vi "Lab Panel V4.85.vi"() -> ()   [LabVIEW 2013] (continued)
                    n2580 = Unbundle(w4668) -> ("DESCRIPTION"=w4648:string)  [unwired: 4 out]
                    n2581 = Unbundle(w4667) -> ("DESCRIPTION"=w4647:string)  [unwired: 4 out]
                    n2582 = Unbundle(w4664) -> ("DESCRIPTION"=w4644:string)  [unwired: 4 out]
                    n2583 = Unbundle(w4670) -> ("DESCRIPTION"=w4650:string)  [unwired: 4 out]
                    n2584 = Unbundle(w4666) -> ("DESCRIPTION"=w4646:string)  [unwired: 4 out]
                    n2585 = Unbundle(w4673) -> ("DESCRIPTION"=w4662:string)  [unwired: 4 out]
                    n2586 = Unbundle(w4671) -> ("DESCRIPTION"=w4651:string)  [unwired: 4 out]
                    n2587 = Unbundle(w4665) -> ("DESCRIPTION"=w4645:string)  [unwired: 4 out]
                    n2588 = Unbundle(w4672) -> ("DESCRIPTION"=w4652:string)  [unwired: 4 out]
                    n2589 = Concatenate Strings("[LAB05-2/", w4644) -> (w4634:string)
                    n2590 = Concatenate Strings("[LAB05-1/", w4645) -> (w4635:string)
                    n2591 = Concatenate Strings("[LAB04-2/", w4646) -> (w4636:string)
                    n2592 = Concatenate Strings("[LAB03-2/", w4648) -> (w4638:string)
                    n2593 = Concatenate Strings("[LAB04-1/", w4647) -> (w4637:string)
                    n2594 = Concatenate Strings("[LAB03-1/", w4649) -> (w4639:string)
                    n2595 = Concatenate Strings("[LAB01-2/", w4652) -> (w4642:string)
                    n2596 = Concatenate Strings("[LAB02-2/", w4650) -> (w4640:string)
                    n2597 = Concatenate Strings("[LAB01-1/", w4662) -> (w4643:string)
                    n2598 = Concatenate Strings("[LAB02-1/", w4651) -> (w4641:string)
                  }
                  frame #1 {
                    w4697 = "/"
                    w4698 = 2.0
                    n2599 = local read "DISP LAB01-2"() -> (w4777:T4)
                    n2600 = local read "DISP LAB01-1"() -> (w4778:T4)
                    n2601 = local read "DISP LAB02-1"() -> (w4776:T4)
                    n2602 = local read "DISP LAB03-2"() -> (w4773:T4)
                    n2603 = local read "DISP LAB02-2"() -> (w4775:T4)
                    n2604 = local read "DISP LAB03-1"() -> (w4774:T4)
                    n2605 = local read "DISP LAB04-2"() -> (w4771:T4)
                    n2606 = local read "DISP LAB04-1"() -> (w4772:T4)
                    n2607 = local read "DISP LAB05-1"() -> (w4770:T4)
                    n2608 = local read "DISP LAB05-2"() -> (w4769:T4)
                    n2609 = Unbundle(w4777) -> ("CYCLE"=w4761:dbl, "MINS"=w4760:dbl, "STATUS"=w4757:string)
                    n2610 = Unbundle(w4778) -> ("CYCLE"=w4766:dbl, "MINS"=w4765:dbl, "STATUS"=w4762:string)
                    n2611 = Unbundle(w4776) -> ("CYCLE"=w4754:dbl, "MINS"=w4753:dbl, "STATUS"=w4752:string)
                    n2612 = Unbundle(w4773) -> ("CYCLE"=w4741:dbl, "MINS"=w4740:dbl, "STATUS"=w4737:string)
                    n2613 = Unbundle(w4774) -> ("CYCLE"=w4746:dbl, "MINS"=w4745:dbl, "STATUS"=w4742:string)
                    n2614 = Unbundle(w4775) -> ("CYCLE"=w4751:dbl, "MINS"=w4750:dbl, "STATUS"=w4747:string)
                    n2615 = Unbundle(w4772) -> ("CYCLE"=w4736:dbl, "MINS"=w4735:dbl, "STATUS"=w4732:string)
                    n2616 = Unbundle(w4771) -> ("CYCLE"=w4731:dbl, "MINS"=w4730:dbl, "STATUS"=w4727:string)
                    n2617 = Unbundle(w4770) -> ("CYCLE"=w4726:dbl, "MINS"=w4725:dbl, "STATUS"=w4722:string)
                    n2618 = Unbundle(w4769) -> ("CYCLE"=w4768:dbl, "MINS"=w4767:dbl, "STATUS"=w4719:string)
                    n2619 = Number To Decimal String(number=w4754) -> (decimal integer string=w4756:string)  [unwired: 1 in]
                    n2620 = Number To Decimal String(number=w4751) -> (decimal integer string=w4749:string)  [unwired: 1 in]
                    n2621 = Number To Decimal String(number=w4746) -> (decimal integer string=w4744:string)  [unwired: 1 in]
                    n2622 = Number To Decimal String(number=w4761) -> (decimal integer string=w4759:string)  [unwired: 1 in]
                    n2623 = Number To Decimal String(number=w4741) -> (decimal integer string=w4739:string)  [unwired: 1 in]
                    n2624 = Number To Decimal String(number=w4766) -> (decimal integer string=w4764:string)  [unwired: 1 in]
                    n2625 = Number To Decimal String(number=w4768) -> (decimal integer string=w4721:string)  [unwired: 1 in]
                    n2626 = Number To Decimal String(number=w4736) -> (decimal integer string=w4734:string)  [unwired: 1 in]
                    n2627 = Number To Decimal String(number=w4731) -> (decimal integer string=w4729:string)  [unwired: 1 in]
                    n2628 = Number To Decimal String(number=w4726) -> (decimal integer string=w4724:string)  [unwired: 1 in]
                    n2629 = Number To Fractional String(number=w4753, precision (6)=w4698) -> (F-format string=w4755:string)  [unwired: 2 in]
                    n2630 = Number To Fractional String(number=w4740, precision (6)=w4698) -> (F-format string=w4738:string)  [unwired: 2 in]
                    n2631 = Number To Fractional String(number=w4750, precision (6)=w4698) -> (F-format string=w4748:string)  [unwired: 2 in]
                    n2632 = Number To Fractional String(number=w4745, precision (6)=w4698) -> (F-format string=w4743:string)  [unwired: 2 in]
                    n2633 = Number To Fractional String(number=w4730, precision (6)=w4698) -> (F-format string=w4728:string)  [unwired: 2 in]
                    n2634 = Number To Fractional String(number=w4735, precision (6)=w4698) -> (F-format string=w4733:string)  [unwired: 2 in]
                    n2635 = Number To Fractional String(number=w4760, precision (6)=w4698) -> (F-format string=w4758:string)  [unwired: 2 in]
                    n2636 = Number To Fractional String(number=w4725, precision (6)=w4698) -> (F-format string=w4723:string)  [unwired: 2 in]
                    n2637 = Number To Fractional String(number=w4765, precision (6)=w4698) -> (F-format string=w4763:string)  [unwired: 2 in]
                    n2638 = Number To Fractional String(number=w4767, precision (6)=w4698) -> (F-format string=w4720:string)  [unwired: 2 in]
                    n2639 = Concatenate Strings(w4697, w4739, w4697, w4738, w4697, w4737) -> (w4713:string)
                    n2640 = Concatenate Strings(w4697, w4734, w4697, w4733, w4697, w4732) -> (w4712:string)
                    n2641 = Concatenate Strings(w4697, w4729, w4697, w4728, w4697, w4727) -> (w4711:string)
                    n2642 = Concatenate Strings(w4697, w4724, w4697, w4723, w4697, w4722) -> (w4710:string)
                    n2643 = Concatenate Strings(w4697, w4721, w4697, w4720, w4697, w4719) -> (w4709:string)
                    n2644 = Concatenate Strings(w4697, w4764, w4697, w4763, w4697, w4762) -> (w4718:string)
                    n2645 = Concatenate Strings(w4697, w4744, w4697, w4743, w4697, w4742) -> (w4714:string)
                    n2646 = Concatenate Strings(w4697, w4759, w4697, w4758, w4697, w4757) -> (w4717:string)
                    n2647 = Concatenate Strings(w4697, w4756, w4697, w4755, w4697, w4752) -> (w4716:string)
                    n2648 = Concatenate Strings(w4697, w4749, w4697, w4748, w4697, w4747) -> (w4715:string)
                    n2649 = Concatenate Strings("]", "\r") -> (w4694:string)
                    n2650 = Concatenate Strings(w4689, w4714, w4694) -> (w4704:string)
                    n2651 = Concatenate Strings(w4691, w4716, w4694) -> (w4706:string)
                    n2652 = Concatenate Strings(w4690, w4715, w4694) -> (w4705:string)
                    n2653 = Concatenate Strings(w4686, w4711, w4694) -> (w4701:string)
                    n2654 = Concatenate Strings(w4687, w4710, w4694) -> (w4702:string)
                    n2655 = Concatenate Strings(w4685, w4712, w4694) -> (w4700:string)
                    n2656 = Concatenate Strings(w4684, w4713, w4694) -> (w4699:string)
                    n2657 = Concatenate Strings(w4688, w4709, w4694) -> (w4703:string)
                    n2658 = Concatenate Strings(w4692, w4717, w4694) -> (w4707:string)
                    n2659 = Concatenate Strings(w4693, w4718, w4694) -> (w4708:string)
                    n2660 = Concatenate Strings(w4708, w4707, w4706, w4705, w4704, w4699, w4700, w4701, w4702, w4703) -> (w4677:string)
                    n2661 = Concatenate Strings("[PANEL/", "DESC/", "CYCLES/", "MINS/", "STATUS]", "\r", w4677) -> (w4676:string)
                    "MAIL REPORT" <- w4676
                    n2662 = global write "Global display 3.vi" "log all"(w4676) -> ()
                  }
                  frame #2 {
                    w4807 = "END"
                    n2663 = local read "mail control"() -> (w4808:string)
                    n2664 = case shown="False" w4803 {
                      tunnel: w4808 -> [w4832 _]
                      tunnel: w4807 -> [w4831 _]
                      tunnel: [w4830 FALSE] -> w4793
                      frame False {
                        n2665 = Equal?(x=w4832, y=w4831) -> (x = y?=w4830:bool)
                      }
                      frame True {
                      }
                    }
                    n2666 = case shown="False" w4809 {
                      tunnel: w4808 -> [w4848 _]
                      tunnel: w4807 -> [w4847 _]
                      tunnel: [w4846 FALSE] -> w4797
                      frame False {
                        n2667 = Equal?(x=w4848, y=w4847) -> (x = y?=w4846:bool)
                      }
                      frame True {
                      }
                    }
                    n2668 = case shown="False" w4806 {
                      tunnel: w4808 -> [w4844 _]
                      tunnel: w4807 -> [w4843 _]
                      tunnel: [w4842 FALSE] -> w4796
                      frame False {
                        n2669 = Equal?(x=w4844, y=w4843) -> (x = y?=w4842:bool)
                      }
                      frame True {
                      }
                    }
                    n2670 = case shown="False" w4804 {
                      tunnel: w4808 -> [w4836 _]
                      tunnel: w4807 -> [w4835 _]
                      tunnel: [w4834 FALSE] -> w4794
                      frame False {
                        n2671 = Equal?(x=w4836, y=w4835) -> (x = y?=w4834:bool)
                      }
                      frame True {
                      }
                    }
                    n2672 = case shown="False" w4805 {
                      tunnel: w4808 -> [w4840 _]
                      tunnel: w4807 -> [w4839 _]
                      tunnel: [w4838 FALSE] -> w4795
                      frame False {
                        n2673 = Equal?(x=w4840, y=w4839) -> (x = y?=w4838:bool)
                      }
                      frame True {
                      }
                    }
                    n2674 = Or(x=w4795, y=w4794) -> (x .or. y?=w4786:bool)
                    n2675 = Or(x=w4797, y=w4796) -> (x .or. y?=w4787:bool)
                    n2676 = Or(x=w4787, y=w4786) -> (x .or. y?=w4782:bool)
                    n2677 = case shown="False" w4799 {
                      tunnel: w4808 -> [w4816 _]
                      tunnel: w4807 -> [w4815 _]
                      tunnel: [w4814 FALSE] -> w4788
                      frame False {
                        n2678 = Equal?(x=w4816, y=w4815) -> (x = y?=w4814:bool)
                      }
                      frame True {
                      }
                    }
                    n2679 = case shown="False" w4798 {
                      tunnel: w4808 -> [w4812 _]
                      tunnel: w4807 -> [w4811 _]
                      tunnel: [w4810 FALSE] -> w4792
                      frame False {
                        n2680 = Equal?(x=w4812, y=w4811) -> (x = y?=w4810:bool)
                      }
                      frame True {
                      }
                    }
                    n2681 = case shown="False" w4800 {
                      tunnel: w4808 -> [w4820 _]
                      tunnel: w4807 -> [w4819 _]
                      tunnel: [w4818 FALSE] -> w4789
                      frame False {
                        n2682 = Equal?(x=w4820, y=w4819) -> (x = y?=w4818:bool)
                      }
                      frame True {
                      }
                    }
                    n2683 = case shown="False" w4802 {
                      tunnel: w4808 -> [w4828 _]
                      tunnel: w4807 -> [w4827 _]
                      tunnel: [w4826 FALSE] -> w4791
                      frame False {
                        n2684 = Equal?(x=w4828, y=w4827) -> (x = y?=w4826:bool)
                      }
                      frame True {
                      }
                    }
                    n2685 = case shown="False" w4801 {
                      tunnel: w4808 -> [w4824 _]
                      tunnel: w4807 -> [w4823 _]
                      tunnel: [w4822 FALSE] -> w4790
                      frame False {
                        n2686 = Equal?(x=w4824, y=w4823) -> (x = y?=w4822:bool)
                      }
                      frame True {
                      }
                    }
                    n2687 = Or(x=w4791, y=w4790) -> (x .or. y?=w4785:bool)
                    n2688 = Or(x=w4789, y=w4788) -> (x .or. y?=w4784:bool)
                    n2689 = Or(x=w4792, y=w4793) -> (x .or. y?=w4780:bool)
                    n2690 = Or(x=w4785, y=w4784) -> (x .or. y?=w4783:bool)
                    n2691 = Or(x=w4782, y=w4783) -> (x .or. y?=w4781:bool)
                    n2692 = Or(x=w4781, y=w4780) -> (x .or. y?=w4779:bool)
                  }
                  frame #3 {
                    n2693 = local read "on loops"() -> (w4862:dbl)
                    n2694 = local read "jig cycle"() -> (w4859:dbl)
                    n2695 = local read "Send Mail Now"() -> (w4853:bool)
                    n2696 = Add(x=w4862, y=3.0) -> (x+y=w4860:dbl)
                    n2697 = Equal?(x=w4859, y=w4860) -> (x = y?=w4854:bool)
                    n2698 = And(x=w4854, y=w4853) -> (x .and. y?=w4852:bool)
                    n2699 = And(x=w4858, y=w4854) -> (x .and. y?=w4857:bool)
                    n2700 = And(x=w4857, y=w4856) -> (x .and. y?=w4855:bool)
                    n2701 = Or(x=w4855, y=w4852) -> (x .or. y?=w4851:bool)
                    n2702 = case shown="True" w4851 {
                      tunnel: w4867 -> [_ w4873]
                      tunnel: w4866 -> [_ w4872]
                      tunnel: "Lab Panel Test Status" -> [_ w4871]
                      tunnel: w4864 -> [_ w4870]
                      tunnel: w4863 -> [_ w4869]
                      tunnel: w4850 -> [_ w4868]
                      frame False {
                      }
                      frame True {
                        n2703 = stacked-sequence {
                          tunnel: w4873 -> [w4881 _]
                          tunnel: w4872 -> [w4880 _]
                          tunnel: w4871 -> [w4879 _]
                          tunnel: w4870 -> [w4878 _]
                          tunnel: w4869 -> [w4877 _]
                          tunnel: w4868 -> [w4876 _]
                          frame #0 {
                            n2704 = call "sub vi - send mail v5.vi"("TO:"=w4881, "subject"=w4879, "from"=w4877, "out going server"=w4878, "message"=w4880) -> ("error out"=w4875:errorcluster)  [unwired: 10 in]
                            n2705 = Bundle(cluster=w4876, "mail error"=w4875) -> (w4874:T6)  [unwired: 6 in]
                            n2706 = local write "MAIL SETTINGS"(w4874) -> ()
                          }
                          frame #1 {
                            n2707 = local write "mail control"("") -> ()
                            n2708 = local write "Send Mail Now"(FALSE) -> ()
                          }
                        }
                      }
                    }
                  }
                }
              }
            }
          }
          frame #18 {
            # "save jig cycle values once all run switches are off"
            n2709 = stacked-sequence {
              tunnel: w4893 -> [_ w4922]
              tunnel: w4892 -> [_ w4921]
              tunnel: w4891 -> [_ w4920]
              tunnel: w4890 -> [_ w4919]
              tunnel: w4889 -> [_ w4918]
              tunnel: w4888 -> [_ w4917]
              tunnel: w4887 -> [_ w4916]
              tunnel: w4886 -> [_ w4915]
              tunnel: w4885 -> [_ w4914]
              tunnel: w4884 -> [_ w4913]
              frame #0 {
              }
              frame #1 {
                n2710 = Not(x=w4913) -> (.not. x?=w4896:bool)
                n2711 = Not(x=w4921) -> (.not. x?=w4911:bool)
                n2712 = Not(x=w4918) -> (.not. x?=w4906:bool)
                n2713 = Not(x=w4916) -> (.not. x?=w4902:bool)
                n2714 = Not(x=w4914) -> (.not. x?=w4898:bool)
                n2715 = Not(x=w4922) -> (.not. x?=w4912:bool)
                n2716 = Not(x=w4920) -> (.not. x?=w4910:bool)
                n2717 = Not(x=w4917) -> (.not. x?=w4904:bool)
                n2718 = Not(x=w4919) -> (.not. x?=w4908:bool)
                n2719 = Not(x=w4915) -> (.not. x?=w4900:bool)
                n2720 = local read "Save JC"() -> (w4924:bool)
                n2721 = And(x=w4912, y=w4911) -> (x .and. y?=w4909:bool)
                n2722 = And(x=w4909, y=w4910) -> (x .and. y?=w4907:bool)
                n2723 = And(x=w4907, y=w4908) -> (x .and. y?=w4905:bool)
                n2724 = And(x=w4905, y=w4906) -> (x .and. y?=w4903:bool)
                n2725 = And(x=w4903, y=w4904) -> (x .and. y?=w4901:bool)
                n2726 = And(x=w4901, y=w4902) -> (x .and. y?=w4899:bool)
                n2727 = And(x=w4899, y=w4900) -> (x .and. y?=w4897:bool)
                n2728 = And(x=w4897, y=w4898) -> (x .and. y?=w4895:bool)
                n2729 = And(x=w4895, y=w4896) -> (x .and. y?=w4894:bool)
                n2730 = And(x=w4894, y=w4924) -> (x .and. y?=w4923:bool)
                n2731 = case shown="True" w4923 {
                  tunnel: w4894 -> [w4925 _]
                  frame False {
                    n2732 = case shown="False" w4925 {
                      frame False {
                        n2733 = local write "Save JC"(TRUE) -> ()
                      }
                      frame True {
                      }
                    }
                  }
                  frame True {
                    n2734 = stacked-sequence {
                      frame #0 {
                        n2735 = String To Path(string="c:\\crabtree\\Jig Cycles\\") -> (path=w4937:path)
                        n2736 = Build Path(base path=w4937, name or relative path="jigcycles.bin") -> (appended path=w4935:path)
                        n2737 = Create Folder(path (use dialog)=w4937) -> (error out=w4939:errorcluster)  [unwired: 2 in, 2 out]
                        n2738 = local read "JIG RELAY CYCLES"() -> (w4929:T7)
                        n2739 = call <vilib>:"Clear Errors.vi"("error in (no error)"=w4939) -> ()  [unwired: 6 in, 1 out]
                        n2740 = local write "Save JC"(FALSE) -> ()
                        n2741 = Open/Create/Replace File(file path (use dialog)=w4935, operation (0:open)=T19."replace or create") -> (refnum out=w4933:refnum<file>, error out=w4934:errorcluster)  [unwired: 4 in, 1 out]
                        n2742 = Write to Binary File(file (use dialog)=w4933, data=w4929, error in=w4934) -> (refnum out=w4932:refnum<file>, error out=w4931:errorcluster)  [unwired: 3 in, 1 out]
                        n2743 = Close File(refnum=w4932, error in=w4931) -> (error out=w4930:errorcluster)  [unwired: 1 out]
                        n2744 = local write "data file error"(w4930) -> ()
                      }
                      frame #1 {
                        n2745 = local read "JIG RELAY CYCLES"() -> (w4962:T7)
                        n2746 = Unbundle By Name(w4962) -> ("LAB01-1"=w4957:dbl, "LAB01-2"=w4956:dbl, "LAB02-1"=w4954:dbl, "LAB02-2"=w4953:dbl, "LAB03-1"=w4951:dbl, "LAB03-2"=w4948:dbl, "LAB04-1"=w4947:dbl, "LAB04-2"=w4945:dbl, "LAB05-1"=w4943:dbl, "LAB05-2"=w4941:dbl)
                        n2747 = stacked-sequence {
                          tunnel: w4957 -> [w4965 _ _ _ _ _ _ _ _ _]
                          tunnel: 1000000 -> [w4968 w4978 w4988 w4998 w5008 w5018 w5028 w5038 w5048 w5058]
                          tunnel: [w4966 _ _ _ _ _ _ _ _ _] -> w4960
                          tunnel: "TEST STATION HAS REACHED 1 MILLION CYCLES, REPLACE  CONTROL RELAYS" -> [w4964 w4976 w4986 w4996 w5006 w5016 w5026 w5036 w5046 w5056]
                          tunnel: [_ w4975 _ _ _ _ _ _ _ _] -> w4958
                          tunnel: w4956 -> [_ w4974 _ _ _ _ _ _ _ _]
                          tunnel: [_ _ w4985 _ _ _ _ _ _ _] -> w4955
                          tunnel: w4954 -> [_ _ w4984 _ _ _ _ _ _ _]
                          tunnel: w4953 -> [_ _ _ w4995 _ _ _ _ _ _]
                          tunnel: [_ _ _ w4994 _ _ _ _ _ _] -> w4952
                          tunnel: w4951 -> [_ _ _ _ w5005 _ _ _ _ _]
                          tunnel: [_ _ _ _ w5004 _ _ _ _ _] -> w4950
                          tunnel: [_ _ _ _ _ w5015 _ _ _ _] -> w4949
                          tunnel: w4948 -> [_ _ _ _ _ w5014 _ _ _ _]
                          tunnel: w4947 -> [_ _ _ _ _ _ w5025 _ _ _]
                          tunnel: [_ _ _ _ _ _ w5024 _ _ _] -> w4946
                          tunnel: w4945 -> [_ _ _ _ _ _ _ w5035 _ _]
                          tunnel: [_ _ _ _ _ _ _ w5034 _ _] -> w4944
                          tunnel: w4943 -> [_ _ _ _ _ _ _ _ w5045 _]
                          tunnel: [_ _ _ _ _ _ _ _ w5044 _] -> w4942
                          tunnel: w4941 -> [_ _ _ _ _ _ _ _ _ w5055]
                          tunnel: [_ _ _ _ _ _ _ _ _ w5054] -> w4940
                          frame #0 {
                            n2748 = Greater?(x=w4965, y=w4968) -> (0:w4967:bool)
                            n2749 = case shown="True" w4967 {
                              tunnel: [w4969 0] -> w4966
                              tunnel: w4965 -> [w4969 _]
                              tunnel: w4964 -> [_ w4970]
                              frame False {
                              }
                              frame True {
                                n2750 = Concatenate Strings("LA01-1 ", w4970) -> (w4973:string)
                                n2751 = One Button Dialog(message=w4973) -> ()  [unwired: 1 in, 1 out]
                              }
                            }
                          }
                          frame #1 {
                            n2752 = Greater?(x=w4974, y=w4978) -> (0:w4977:bool)
                            n2753 = case shown="True" w4977 {
                              tunnel: [w4979 0] -> w4975
                              tunnel: w4974 -> [w4979 _]
                              tunnel: w4976 -> [_ w4980]
                              frame False {
                              }
                              frame True {
                                n2754 = Concatenate Strings("LA01-2 ", w4980) -> (w4983:string)
                                n2755 = One Button Dialog(message=w4983) -> ()  [unwired: 1 in, 1 out]
                              }
                            }
                          }
                          frame #2 {
                            n2756 = Greater?(x=w4984, y=w4988) -> (0:w4987:bool)
                            n2757 = case shown="True" w4987 {
                              tunnel: [w4989 0] -> w4985
                              tunnel: w4984 -> [w4989 _]
                              tunnel: w4986 -> [_ w4990]
                              frame False {
                              }
                              frame True {
                                n2758 = Concatenate Strings("LA02-1 ", w4990) -> (w4993:string)
                                n2759 = One Button Dialog(message=w4993) -> ()  [unwired: 1 in, 1 out]
                              }
                            }
                          }
                          frame #3 {
                            n2760 = Greater?(x=w4995, y=w4998) -> (0:w4997:bool)
                            n2761 = case shown="True" w4997 {
                              tunnel: [w4999 0] -> w4994
                              tunnel: w4995 -> [w4999 _]
                              tunnel: w4996 -> [_ w5000]
                              frame False {
                              }
                              frame True {
                                n2762 = Concatenate Strings("LA02-2 ", w5000) -> (w5003:string)
                                n2763 = One Button Dialog(message=w5003) -> ()  [unwired: 1 in, 1 out]
                              }
                            }
                          }
                          frame #4 {
                            n2764 = Greater?(x=w5005, y=w5008) -> (0:w5007:bool)
                            n2765 = case shown="True" w5007 {
                              tunnel: [w5009 0] -> w5004
                              tunnel: w5005 -> [w5009 _]
                              tunnel: w5006 -> [_ w5010]
                              frame False {
                              }
                              frame True {
                                n2766 = Concatenate Strings("LA03-1 ", w5010) -> (w5013:string)
                                n2767 = One Button Dialog(message=w5013) -> ()  [unwired: 1 in, 1 out]
                              }
                            }
                          }
                          frame #5 {
                            n2768 = Greater?(x=w5014, y=w5018) -> (0:w5017:bool)
                            n2769 = case shown="True" w5017 {
                              tunnel: [w5019 0] -> w5015
                              tunnel: w5014 -> [w5019 _]
                              tunnel: w5016 -> [_ w5020]
                              frame False {
                              }
                              frame True {
                                n2770 = Concatenate Strings("LA03-2 ", w5020) -> (w5023:string)
                                n2771 = One Button Dialog(message=w5023) -> ()  [unwired: 1 in, 1 out]
                              }
                            }
                          }
                          frame #6 {
                            n2772 = Greater?(x=w5025, y=w5028) -> (0:w5027:bool)
                            n2773 = case shown="True" w5027 {
                              tunnel: [w5029 0] -> w5024
                              tunnel: w5025 -> [w5029 _]
                              tunnel: w5026 -> [_ w5030]
                              frame False {
                              }
                              frame True {
                                n2774 = Concatenate Strings("LA04-1 ", w5030) -> (w5033:string)
                                n2775 = One Button Dialog(message=w5033) -> ()  [unwired: 1 in, 1 out]
                              }
                            }
                          }
                          frame #7 {
                            n2776 = Greater?(x=w5035, y=w5038) -> (0:w5037:bool)
                            n2777 = case shown="True" w5037 {
                              tunnel: [w5039 0] -> w5034
                              tunnel: w5035 -> [w5039 _]
                              tunnel: w5036 -> [_ w5040]
                              frame False {
                              }
                              frame True {
                                n2778 = Concatenate Strings("LA04-2 ", w5040) -> (w5043:string)
                                n2779 = One Button Dialog(message=w5043) -> ()  [unwired: 1 in, 1 out]
                              }
                            }
                          }
                          frame #8 {
                            n2780 = Greater?(x=w5045, y=w5048) -> (0:w5047:bool)
                            n2781 = case shown="True" w5047 {
                              tunnel: [w5049 0] -> w5044
                              tunnel: w5045 -> [w5049 _]
                              tunnel: w5046 -> [_ w5050]
                              frame False {
                              }
                              frame True {
                                n2782 = Concatenate Strings("LA05-1 ", w5050) -> (w5053:string)
                                n2783 = One Button Dialog(message=w5053) -> ()  [unwired: 1 in, 1 out]
                              }
                            }
                          }
                          frame #9 {
                            n2784 = Greater?(x=w5055, y=w5058) -> (0:w5057:bool)
                            n2785 = case shown="True" w5057 {
                              tunnel: [w5059 0] -> w5054
                              tunnel: w5055 -> [w5059 _]
                              tunnel: w5056 -> [_ w5060]
                              frame False {
                              }
                              frame True {
                                n2786 = Concatenate Strings("LA05-2 ", w5060) -> (w5063:string)
                                n2787 = One Button Dialog(message=w5063) -> ()  [unwired: 1 in, 1 out]
                              }
                            }
                          }
                        }
                        n2788 = Bundle By Name(cluster=w4962, "LAB01-1"=w4960, "LAB01-2"=w4958, "LAB02-1"=w4955, "LAB02-2"=w4952, "LAB03-1"=w4950, "LAB03-2"=w4949, "LAB04-1"=w4946, "LAB04-2"=w4944, "LAB05-1"=w4942, "LAB05-2"=w4940) -> (w4961:T7)
                        n2789 = local write "JIG RELAY CYCLES"(w4961) -> ()
                      }
                    }
                  }
                }
              }
            }
          }
          frame #19 {
            # "get temperature values"
            n2790 = local read "simulate"() -> (w5076:bool)
            n2791 = local read "Temp Test Cal"() -> (w5073:dbl)
            n2792 = stacked-sequence {
              tunnel: w5076 -> [_ w5132 w5177 w5222 w5267 w5312]
              tunnel: T12 {"1  (A) cal"=1.0, "1 (V) cal"=1.0, "1 (PF) cal"=1.0, "1 (TL) cal"=1.0, "1 (TN) cal"=1.0, "2 (A) cal"=1.0, "2 (V) cal"=1.0, "2 (PF) cal"=1.0, "2 (TL) cal"=1.0, "2 (TN) cal"=1.0} ("CAL LAB01") -> [_ w5131 w5176 w5221 w5266 w5311]
              tunnel: w5074 -> [_ w5129 _ _ _ _]
              tunnel: w5073 -> [_ w5125 w5175 w5220 w5265 w5310]
              tunnel: w5072 -> [_ w5120 _ _ _ _]
              tunnel: w5071 -> [_ _ w5166 _ _ _]
              tunnel: w5070 -> [_ _ w5165 _ _ _]
              tunnel: w5069 -> [_ _ _ w5211 _ _]
              tunnel: w5068 -> [_ _ _ w5210 _ _]
              tunnel: w5067 -> [_ _ _ _ w5256 _]
              tunnel: w5066 -> [_ _ _ _ w5255 _]
              tunnel: w5065 -> [_ _ _ _ _ w5301]
              tunnel: w5064 -> [_ _ _ _ _ w5300]
              frame #0 {
                n2793 = local read "Select COM port"() -> (w5081:refnum<visa-resource-name>)
                "COM port" <- w5081
                n2794 = local read "jig cycle"() -> (w5082:dbl)
                n2795 = local read "on loops"() -> (w5084:dbl)
                n2796 = global write "Global 1.vi" "tmp dly lps"("Temp Delay Lps") -> ()
                n2797 = global write "Global 1.vi" "dly value"("Temp Value") -> ()
                n2798 = Add(x=w5084, y=3) -> (x+y=w5085:dbl)
                n2799 = global write "Global 1.vi" "COM port"(w5081) -> ()
                n2800 = Equal?(x=w5082, y=w5085) -> (x = y?=w5078:bool)
                n2801 = local read "Temp Loops"() -> (w5077:dbl)
                n2802 = case shown="True" w5078 {
                  tunnel: w5077 -> [_ w5087]
                  frame False {
                  }
                  frame True {
                    n2803 = stacked-sequence {
                      tunnel: w5087 -> [w5090 w5118]
                      frame #0 {
                        n2804 = local read "simulate"() -> (w5088:bool)
                        n2805 = case shown="5" w5090 {
                          tunnel: 1.0 -> [_ w5095 w5097 w5103 w5107 w5112]
                          tunnel: w5088 -> [_ w5091 w5096 w5101 w5108 w5111]
                          frame 0, Default {
                          }
                          frame 1 {
                            w5093 = FALSE
                            n2806 = call "sub vi - GET ALL TEMP v5.vi"("LA01-EN"=TRUE, "simulate"=w5091, "LA02-EN"=w5093, "LA03-EN"=w5093, "LA04-EN"=w5093, "LA05-EN"=w5093, "Gen Cal Value"=w5095) -> ("LA01 TEMP"=w5092:T22)  [unwired: 3 in, 5 out]
                            n2807 = local write "LAB01 TEMP"(w5092) -> ()
                          }
                          frame 2 {
                            w5098 = FALSE
                            n2808 = call "sub vi - GET ALL TEMP v5.vi"("LA01-EN"=w5098, "simulate"=w5096, "LA02-EN"=TRUE, "LA03-EN"=w5098, "LA04-EN"=w5098, "LA05-EN"=w5098, "Gen Cal Value"=w5097) -> ("LA02 TEMP"=w5100:T22)  [unwired: 3 in, 5 out]
                            n2809 = local write "LAB02 TEMP"(w5100) -> ()
                          }
                          frame 3 {
                            w5104 = FALSE
                            n2810 = call "sub vi - GET ALL TEMP v5.vi"("LA01-EN"=w5104, "simulate"=w5101, "LA02-EN"=w5104, "LA03-EN"=TRUE, "LA04-EN"=w5104, "LA05-EN"=w5104, "Gen Cal Value"=w5103) -> ("LA03 TEMP"=w5102:T22)  [unwired: 3 in, 5 out]
                            n2811 = local write "LAB03 TEMP"(w5102) -> ()
                          }
                          frame 4 {
                            w5109 = FALSE
                            n2812 = call "sub vi - GET ALL TEMP v5.vi"("LA01-EN"=w5109, "simulate"=w5108, "LA02-EN"=w5109, "LA03-EN"=w5109, "LA04-EN"=TRUE, "LA05-EN"=w5109, "Gen Cal Value"=w5107) -> ("LA04 TEMP"=w5106:T22)  [unwired: 3 in, 5 out]
                            n2813 = local write "LAB04 TEMP"(w5106) -> ()
                          }
                          frame 5 {
                            w5114 = FALSE
                            n2814 = call "sub vi - GET ALL TEMP v5.vi"("LA01-EN"=w5114, "simulate"=w5111, "LA02-EN"=w5114, "LA03-EN"=w5114, "LA04-EN"=w5114, "LA05-EN"=TRUE, "Gen Cal Value"=w5112) -> ("LA05 TEMP"=w5113:T22)  [unwired: 3 in, 5 out]
                            n2815 = local write "LAB05 TEMP"(w5113) -> ()
                          }
                        }
                      }
                      frame #1 {
                        n2816 = Greater Or Equal?(x=w5118, y=5) -> (x >= y?=w5116:bool)
                        n2817 = case shown="True" w5116 {
                          frame False {
                          }
                          frame True {
                            n2818 = local write "Temp Loops"(0) -> ()
                          }
                        }
                      }
                    }
                    n2819 = local write "TEMP"(TRUE) -> ()
                  }
                }
              }
              frame #1 {
                n2820 = case shown="False" w5132 {
                  tunnel: [w5163 w5164] -> w5148
                  tunnel: w5131 -> [_ w5164]
                  frame False {
                    n2821 = local read "CAL LAB01"() -> (w5163:T12)
                  }
                  frame True {
                  }
                }
                n2822 = local read "LAB01 TEMP"() -> (w5138:T11)
                n2823 = local read "TEMP LA01"() -> (w5139:T8)
                n2824 = call "sub vi - temperature delay v2.vi"("temp values IN"=w5139, "temp signals"=w5138) -> ("T2-N"=w5134:dbl, "T2-L"=w5135:dbl, "T1-N"=w5136:dbl, "T1-L"=w5137:dbl, "temp values OUT"=w5133:T40)  [unwired: 5 in]
                n2825 = Unbundle By Name(w5148) -> ("1 (TL) cal"=w5143:dbl, "1 (TN) cal"=w5142:dbl, "2 (TL) cal"=w5141:dbl, "2 (TN) cal"=w5140:dbl)  [unwired: 6 out]
                n2826 = local write "TEMP LA01"(w5133) -> ()
                n2827 = Multiply(x=w5137, y=w5143) -> (x*y=w5130:dbl)
                n2828 = Multiply(x=w5136, y=w5142) -> (x*y=w5127:dbl)
                n2829 = Multiply(x=w5135, y=w5141) -> (x*y=w5124:dbl)
                n2830 = Multiply(x=w5134, y=w5140) -> (x*y=w5123:dbl)
                n2831 = case shown="True" w5129 {
                  tunnel: w5130 -> [w5157 w5162]
                  tunnel: w5125 -> [_ w5160]
                  tunnel: [w5157 w5161] -> w5128
                  tunnel: w5127 -> [w5156 w5159]
                  tunnel: [w5156 w5158] -> w5126
                  frame False {
                  }
                  frame True {
                    n2832 = Multiply(x=w5160, y=w5159) -> (x*y=w5158:dbl)
                    n2833 = Multiply(x=w5160, y=w5162) -> (x*y=w5161:dbl)
                  }
                }
                n2834 = case shown="True" w5120 {
                  tunnel: w5124 -> [w5150 w5155]
                  tunnel: w5125 -> [_ w5153]
                  tunnel: [w5150 w5154] -> w5122
                  tunnel: w5123 -> [w5149 w5152]
                  tunnel: [w5149 w5151] -> w5121
                  frame False {
                  }
                  frame True {
                    n2835 = Multiply(x=w5153, y=w5152) -> (x*y=w5151:dbl)
                    n2836 = Multiply(x=w5153, y=w5155) -> (x*y=w5154:dbl)
                  }
                }
                n2837 = local read "SIG LAB01-2"() -> (w5145:T2)
                n2838 = local read "SIG LAB01-1"() -> (w5147:T2)
                n2839 = Bundle By Name(cluster=w5147, "Tmp Live"=w5128, "Tmp Neut"=w5126) -> (w5146:T2)
                n2840 = Bundle By Name(cluster=w5145, "Tmp Live"=w5122, "Tmp Neut"=w5121) -> (w5144:T2)
                n2841 = local write "SIG LAB01-1"(w5146) -> ()
                n2842 = local write "SIG LAB01-2"(w5144) -> ()
              }
              frame #2 {
                n2843 = case shown="True" w5177 {
                  tunnel: [w5208 w5209] -> w5193
                  tunnel: w5176 -> [_ w5209]
                  frame False {
                    n2844 = local read "CAL LAB02"() -> (w5208:T13)
                  }
                  frame True {
                  }
                }
                n2845 = local read "LAB02 TEMP"() -> (w5184:T11)
                n2846 = local read "TEMP LA02"() -> (w5183:T8)
                n2847 = call "sub vi - temperature delay v2.vi"("temp values IN"=w5183, "temp signals"=w5184) -> ("T2-N"=w5178:dbl, "T2-L"=w5179:dbl, "T1-N"=w5180:dbl, "T1-L"=w5181:dbl, "temp values OUT"=w5182:T40)  [unwired: 5 in]
                n2848 = Unbundle By Name(w5193) -> ("1 (TL) cal"=w5188:dbl, "1 (TN) cal"=w5187:dbl, "2 (TL) cal"=w5186:dbl, "2 (TN) cal"=w5185:dbl)  [unwired: 6 out]
                n2849 = local write "TEMP LA02"(w5182) -> ()
                n2850 = Multiply(x=w5181, y=w5188) -> (x*y=w5174:dbl)
                n2851 = Multiply(x=w5180, y=w5187) -> (x*y=w5173:dbl)
                n2852 = Multiply(x=w5179, y=w5186) -> (x*y=w5170:dbl)
                n2853 = Multiply(x=w5178, y=w5185) -> (x*y=w5169:dbl)
                n2854 = case shown="True" w5166 {
                  tunnel: w5174 -> [w5202 w5207]
                  tunnel: w5175 -> [_ w5205]
                  tunnel: [w5202 w5206] -> w5172
                  tunnel: w5173 -> [w5201 w5204]
                  tunnel: [w5201 w5203] -> w5171
                  frame False {
                  }
                  frame True {
                    n2855 = Multiply(x=w5205, y=w5204) -> (x*y=w5203:dbl)
                    n2856 = Multiply(x=w5205, y=w5207) -> (x*y=w5206:dbl)
                  }
                }
                n2857 = case shown="True" w5165 {
                  tunnel: w5170 -> [w5195 w5200]
                  tunnel: w5175 -> [_ w5198]
                  tunnel: [w5195 w5199] -> w5168
                  tunnel: w5169 -> [w5194 w5197]
                  tunnel: [w5194 w5196] -> w5167
                  frame False {
                  }
                  frame True {
                    n2858 = Multiply(x=w5198, y=w5197) -> (x*y=w5196:dbl)
                    n2859 = Multiply(x=w5198, y=w5200) -> (x*y=w5199:dbl)
                  }
                }
                n2860 = local read "SIG LAB02-2"() -> (w5190:T2)
                n2861 = local read "SIG LAB02-1"() -> (w5192:T2)
                n2862 = Bundle By Name(cluster=w5192, "Tmp Live"=w5172, "Tmp Neut"=w5171) -> (w5191:T2)
                n2863 = Bundle By Name(cluster=w5190, "Tmp Live"=w5168, "Tmp Neut"=w5167) -> (w5189:T2)
                n2864 = local write "SIG LAB02-1"(w5191) -> ()
                n2865 = local write "SIG LAB02-2"(w5189) -> ()
              }
              frame #3 {
                n2866 = case shown="False" w5222 {
                  tunnel: [w5253 w5254] -> w5238
                  tunnel: w5221 -> [_ w5254]
                  frame False {
                    n2867 = local read "CAL LAB03"() -> (w5253:T12)
                  }
                  frame True {
                  }
                }
                n2868 = local read "TEMP LA03"() -> (w5228:T8)
                n2869 = local read "LAB03 TEMP"() -> (w5229:T11)
                n2870 = call "sub vi - temperature delay v2.vi"("temp values IN"=w5228, "temp signals"=w5229) -> ("T2-N"=w5223:dbl, "T2-L"=w5224:dbl, "T1-N"=w5225:dbl, "T1-L"=w5226:dbl, "temp values OUT"=w5227:T40)  [unwired: 5 in]
                n2871 = Unbundle By Name(w5238) -> ("1 (TL) cal"=w5233:dbl, "1 (TN) cal"=w5232:dbl, "2 (TL) cal"=w5231:dbl, "2 (TN) cal"=w5230:dbl)  [unwired: 6 out]
                n2872 = local write "TEMP LA03"(w5227) -> ()
                n2873 = Multiply(x=w5226, y=w5233) -> (x*y=w5219:dbl)
                n2874 = Multiply(x=w5225, y=w5232) -> (x*y=w5218:dbl)
                n2875 = Multiply(x=w5224, y=w5231) -> (x*y=w5215:dbl)
                n2876 = Multiply(x=w5223, y=w5230) -> (x*y=w5214:dbl)
                n2877 = case shown="True" w5210 {
                  tunnel: w5215 -> [w5240 w5245]
                  tunnel: w5220 -> [_ w5243]
                  tunnel: [w5240 w5244] -> w5213
                  tunnel: w5214 -> [w5239 w5242]
                  tunnel: [w5239 w5241] -> w5212
                  frame False {
                  }
                  frame True {
                    n2878 = Multiply(x=w5243, y=w5242) -> (x*y=w5241:dbl)
                    n2879 = Multiply(x=w5243, y=w5245) -> (x*y=w5244:dbl)
                  }
                }
                n2880 = case shown="True" w5211 {
                  tunnel: w5219 -> [w5247 w5252]
                  tunnel: w5220 -> [_ w5250]
                  tunnel: [w5247 w5251] -> w5217
                  tunnel: w5218 -> [w5246 w5249]
                  tunnel: [w5246 w5248] -> w5216
                  frame False {
                  }
                  frame True {
                    n2881 = Multiply(x=w5250, y=w5249) -> (x*y=w5248:dbl)
                    n2882 = Multiply(x=w5250, y=w5252) -> (x*y=w5251:dbl)
                  }
                }
                n2883 = local read "SIG LAB03-2"() -> (w5235:T2)
                n2884 = local read "SIG LAB03-1"() -> (w5237:T2)
                n2885 = Bundle By Name(cluster=w5237, "Tmp Live"=w5217, "Tmp Neut"=w5216) -> (w5236:T2)
                n2886 = Bundle By Name(cluster=w5235, "Tmp Live"=w5213, "Tmp Neut"=w5212) -> (w5234:T2)
                n2887 = local write "SIG LAB03-1"(w5236) -> ()
                n2888 = local write "SIG LAB03-2"(w5234) -> ()
              }
              frame #4 {
                n2889 = case shown="False" w5267 {
                  tunnel: [w5298 w5299] -> w5283
                  tunnel: w5266 -> [_ w5299]
                  frame False {
                    n2890 = local read "CAL LAB04"() -> (w5298:T12)
                  }
                  frame True {
                  }
                }
                n2891 = local read "LAB04 TEMP"() -> (w5273:T11)
                n2892 = local read "TEMP LA04"() -> (w5274:T8)
                n2893 = call "sub vi - temperature delay v2.vi"("temp values IN"=w5274, "temp signals"=w5273) -> ("T2-N"=w5268:dbl, "T2-L"=w5269:dbl, "T1-N"=w5270:dbl, "T1-L"=w5271:dbl, "temp values OUT"=w5272:T40)  [unwired: 5 in]
                n2894 = Unbundle By Name(w5283) -> ("1 (TL) cal"=w5278:dbl, "1 (TN) cal"=w5277:dbl, "2 (TL) cal"=w5276:dbl, "2 (TN) cal"=w5275:dbl)  [unwired: 6 out]
                n2895 = local write "TEMP LA04"(w5272) -> ()
                n2896 = Multiply(x=w5271, y=w5278) -> (x*y=w5264:dbl)
                n2897 = Multiply(x=w5270, y=w5277) -> (x*y=w5263:dbl)
                n2898 = Multiply(x=w5269, y=w5276) -> (x*y=w5260:dbl)
                n2899 = Multiply(x=w5268, y=w5275) -> (x*y=w5259:dbl)
                n2900 = case shown="True" w5255 {
                  tunnel: w5260 -> [w5285 w5290]
                  tunnel: w5265 -> [_ w5288]
                  tunnel: [w5285 w5289] -> w5258
                  tunnel: w5259 -> [w5284 w5287]
                  tunnel: [w5284 w5286] -> w5257
                  frame False {
                  }
                  frame True {
                    n2901 = Multiply(x=w5288, y=w5287) -> (x*y=w5286:dbl)
                    n2902 = Multiply(x=w5288, y=w5290) -> (x*y=w5289:dbl)
                  }
                }
                n2903 = case shown="True" w5256 {
                  tunnel: w5264 -> [w5292 w5297]
                  tunnel: w5265 -> [_ w5295]
                  tunnel: [w5292 w5296] -> w5262
                  tunnel: w5263 -> [w5291 w5294]
                  tunnel: [w5291 w5293] -> w5261
                  frame False {
                  }
                  frame True {
                    n2904 = Multiply(x=w5295, y=w5294) -> (x*y=w5293:dbl)
                    n2905 = Multiply(x=w5295, y=w5297) -> (x*y=w5296:dbl)
                  }
                }
                n2906 = local read "SIG LAB04-2"() -> (w5280:T2)
                n2907 = local read "SIG LAB04-1"() -> (w5282:T2)
                n2908 = Bundle By Name(cluster=w5282, "Tmp Live"=w5262, "Tmp Neut"=w5261) -> (w5281:T2)
                n2909 = Bundle By Name(cluster=w5280, "Tmp Live"=w5258, "Tmp Neut"=w5257) -> (w5279:T2)
                n2910 = local write "SIG LAB04-1"(w5281) -> ()
                n2911 = local write "SIG LAB04-2"(w5279) -> ()
              }
              frame #5 {
                n2912 = case shown="False" w5312 {
                  tunnel: [w5343 w5344] -> w5328
                  tunnel: w5311 -> [_ w5344]
                  frame False {
                    n2913 = local read "CAL LAB05"() -> (w5343:T12)
                  }
                  frame True {
                  }
                }
                n2914 = local read "LAB05 TEMP"() -> (w5318:T11)
                n2915 = local read "TEMP LA05"() -> (w5319:T8)
                n2916 = call "sub vi - temperature delay v2.vi"("temp values IN"=w5319, "temp signals"=w5318) -> ("T2-N"=w5314:dbl, "T2-L"=w5315:dbl, "T1-N"=w5316:dbl, "T1-L"=w5317:dbl, "temp values OUT"=w5313:T40)  [unwired: 5 in]
                n2917 = local write "TEMP LA05"(w5313) -> ()
                n2918 = Unbundle By Name(w5328) -> ("1 (TL) cal"=w5320:dbl, "1 (TN) cal"=w5323:dbl, "2 (TL) cal"=w5322:dbl, "2 (TN) cal"=w5321:dbl)  [unwired: 6 out]
                n2919 = Multiply(x=w5317, y=w5320) -> (x*y=w5309:dbl)
                n2920 = Multiply(x=w5316, y=w5323) -> (x*y=w5308:dbl)
                n2921 = Multiply(x=w5315, y=w5322) -> (x*y=w5305:dbl)
                n2922 = Multiply(x=w5314, y=w5321) -> (x*y=w5304:dbl)
                n2923 = case shown="True" w5300 {
                  tunnel: w5305 -> [w5330 w5335]
                  tunnel: w5310 -> [_ w5333]
                  tunnel: [w5330 w5334] -> w5303
                  tunnel: w5304 -> [w5329 w5332]
                  tunnel: [w5329 w5331] -> w5302
                  frame False {
                  }
                  frame True {
                    n2924 = Multiply(x=w5333, y=w5332) -> (x*y=w5331:dbl)
                    n2925 = Multiply(x=w5333, y=w5335) -> (x*y=w5334:dbl)
                  }
                }
                n2926 = case shown="True" w5301 {
                  tunnel: w5309 -> [w5337 w5342]
                  tunnel: w5310 -> [_ w5340]
                  tunnel: [w5337 w5341] -> w5307
                  tunnel: w5308 -> [w5336 w5339]
                  tunnel: [w5336 w5338] -> w5306
                  frame False {
                  }
